vi "Obtain Message Queue.vi"(8 "error in (no error)":errorcluster) -> (0 "error out":errorcluster, 3 "Message Queue out":refnum<queue>)   [LabVIEW 2016, in "Message Queue.lvlib"]
uses:
  Message Queue.lvlib
  Message.ctl
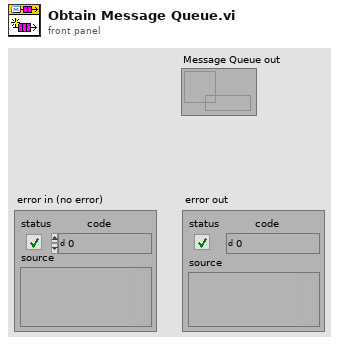
[diagram p1: front panel]
types:
  T1 = typedef "Message Queue.lvlib/Message.ctl" = cluster{"State":string, "Data":variant}
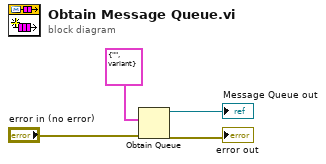
[diagram p0: block diagram]
diagram:
  n1 = Obtain Queue(element data type=T1 {"State"="", "Data"=variant} ("Message"), error in (no error)="error in (no error)") -> (queue out=→"Message Queue out":refnum<queue>, error out=→"error out":errorcluster)  [unwired: 3 in, 1 out]
